vi "Remove_Spikes_sub.vi"(6 "Spikes Array In":cluster{"Index":i32, "max value":dbl}[](array[cluster]), 8 "Number of Sigma to cut after":dbl=3.0, 9 "Number of samples":i32, 10 "Time Trace in":dbl[](array[numeric]), 11 "Bkgnd Variance":dbl) -> (0 "Checked":bool, 2 "Time Trace out":dbl[](array[numeric]), 4 "Spikes Array Out":cluster{"Index":i32, "max value":dbl}[](array[cluster]))   [LabVIEW 2018]
uses:
  <vilib>/Analysis/NI_AALBase.lvlib
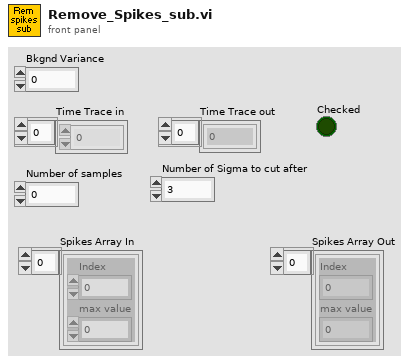
[diagram p1: front panel]
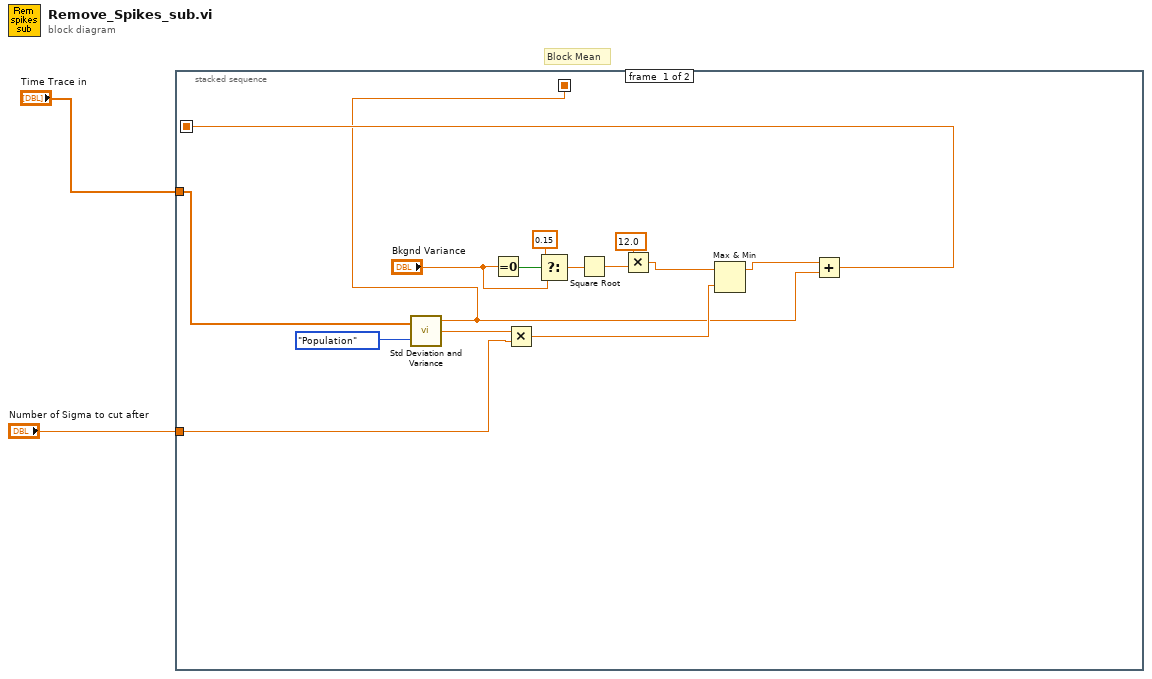
[diagram p0: block diagram]
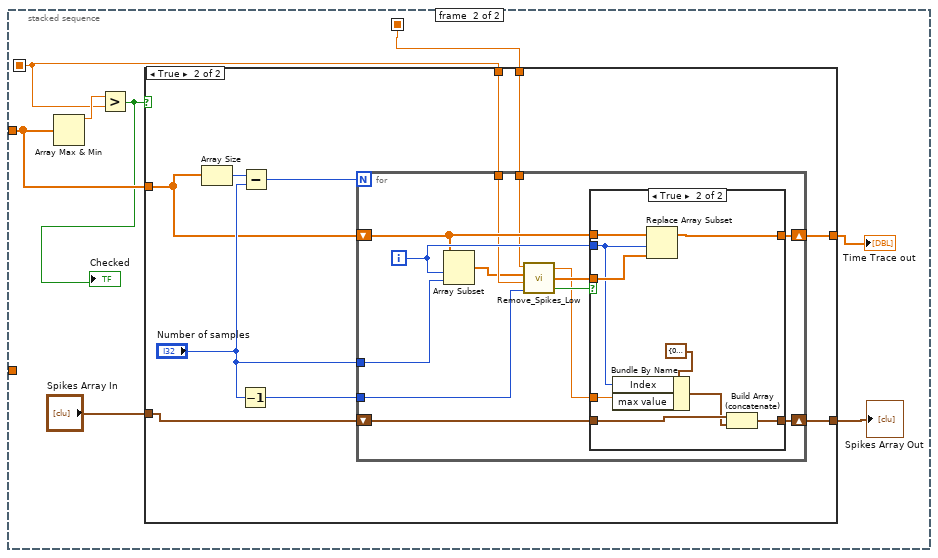
[diagram p2: hidden frame]
diagram:
  # "Block Mean"
  n1 = stacked-sequence {
    seq-local: [w10 _] -> [_ w22]
    seq-local: [w3 _] -> [_ w18]
    tunnel: "Time Trace in" -> [w11 w23]
    tunnel: "Number of Sigma to cut after" -> [w4 _]
    frame #0 {
      n2 = call <vilib>:"Std Deviation and Variance.vi"("X"=w11, "Weighting (Sample)"=enum16{"Sample", "Population"}."Population") -> ("mean"=w3:dbl, "standard deviation"=w8:dbl)  [unwired: 1 out]
      n3 = Equal To 0?(x="Bkgnd Variance") -> (x = 0?=w17:bool)
      n4 = Multiply(x=w8, y=w4) -> (x*y=w6:dbl)
      n5 = Select(t=0.15, s=w17, f="Bkgnd Variance") -> (s? t:f=w15:dbl)
      n6 = Square Root(x=w15) -> (sqrt(x)=w13:dbl)
      n7 = Multiply(x=12.0 ("y"), y=w13) -> (x*y=w7:dbl)
      n8 = Max & Min(x=w7, y=w6) -> (max(x,y)=w5:dbl)  [unwired: 1 out]
      n9 = Add(x=w5, y=w3) -> (x+y=w10:dbl)
    }
    frame #1 {
      n10 = Array Max & Min(array=w23) -> (max value=w24:dbl)  [unwired: 3 out]
      n11 = Greater?(x=w24, y=w22) -> (0:w21:bool)
      "Checked" <- w21
      n12 = case shown="True" w21 {
        tunnel: [w26 w36] -> w20
        tunnel: [w27 w35] -> w25
        tunnel: w22 -> [_ w31]
        tunnel: w23 -> [w27 w30]
        tunnel: "Spikes Array In" -> [w26 w29]
        tunnel: w18 -> [_ w28]
        frame False {
        }
        frame True {
          n13 = Array Size(array=w30) -> (size(s)=w33:i32)
          n14 = Decrement(x="Number of samples") -> (x-1=w32:i32)
          n15 = Subtract(x=w33, y="Number of samples") -> (x-y=w34:i32)
          n16 = for {
            N: w34 -> [_]
            shift-right: [w44] -> w35
            shift-left: w30 -> [w45]
            tunnel: "Number of samples" -> [w50]
            tunnel: w32 -> [w49]
            tunnel: w31 -> [w43]
            shift-right: [w42] -> w36
            shift-left: w29 -> [w41]
            tunnel: w28 -> [w38]
            i -> [w47]
            n17 = Array Subset(array=w45, index=w47, length=w50) -> (w40:dbl[])
            n18 = call "Remove_Spikes_Low.vi"("index"=w49, "Background noise"=w43, "Time Trace"=w40, "Block Mean"=w38) -> ("Spike"=w48:bool, "Filtered Time Trace"=w46:dbl[], "max value"=w39:dbl)
            n19 = case shown="True" w48 {
              tunnel: w47 -> [_ w58]
              tunnel: w46 -> [_ w61]
              tunnel: w45 -> [w52 w60]
              tunnel: [w52 w59] -> w44
              tunnel: [w51 w55] -> w42
              tunnel: w41 -> [w51 w56]
              tunnel: w39 -> [_ w57]
              frame False {
              }
              frame True {
                n20 = Bundle By Name(cluster=cluster{"Index":i32, "max value":dbl} {"Index"=0, "max value"=0.0} ("output cluster"), "Index"=w58, "max value"=w57) -> (w54:cluster{"Index":i32, "max value":dbl})
                n21 = Replace Array Subset(array=w60, new element=w61, index=w58) -> (w59:dbl[])
                n22 = Build Array (concatenate)(w56, w54) -> (w55:cluster{"Index":i32, "max value":dbl}[])
              }
            }
          }
        }
      }
      "Time Trace out" <- w25
      "Spikes Array Out" <- w20
    }
  }
